vi "g_Excel Attributes.vi"() -> ()   [LabVIEW 2015, in "Admin_Actor.lvlib" / "ExcelReader.lvclass"]
uses:
  ExcelReader.lvclass
panel:
  in  "size_Data":cluster{"Row":i32, "Column":i32}={"Row"=7, "Column"=6}
  in  "pos_Data":cluster{"Row":i32, "Column":i32}={"Row"=12, "Column"=1}
  in  "size_table":cluster{"Row":i32, "Column":i32}={"Row"=19, "Column"=7}
  in  "pos_Department":cluster{"Row":i32, "Column":i32}={"Row"=3, "Column"=1}
  in  "pos_Name":cluster{"Row":i32, "Column":i32}={"Row"=3, "Column"=9}
  in  "pos_Date":cluster{"Row":i32, "Column":i32}={"Row"=4, "Column"=1}
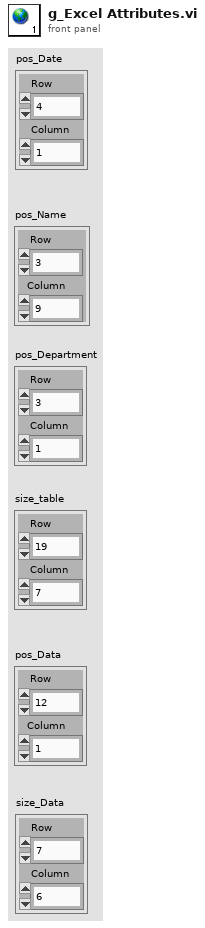
[diagram p1: front panel]
diagram:
